vi "Check Overlay Settings.vi"(8 "error in (no error)":errorcluster, 9 "Mode":T2(ring), 10 "Overlay Settings":T3, 11 "Refnum in":T4) -> (0 "error out":errorcluster, 2 "Report Data":T1, 3 "Refnum out":T4)   [LabVIEW 2015]
uses:
  <vilib>/vision/Image Controls.llb/IMAQ Image.ctl
  Typedef/Last Mouse Position.ctl
  Typedef/Report Data.ctl
panel:
  out "accurate":dbl
  out "Dist.":dbl[][](array[numeric])
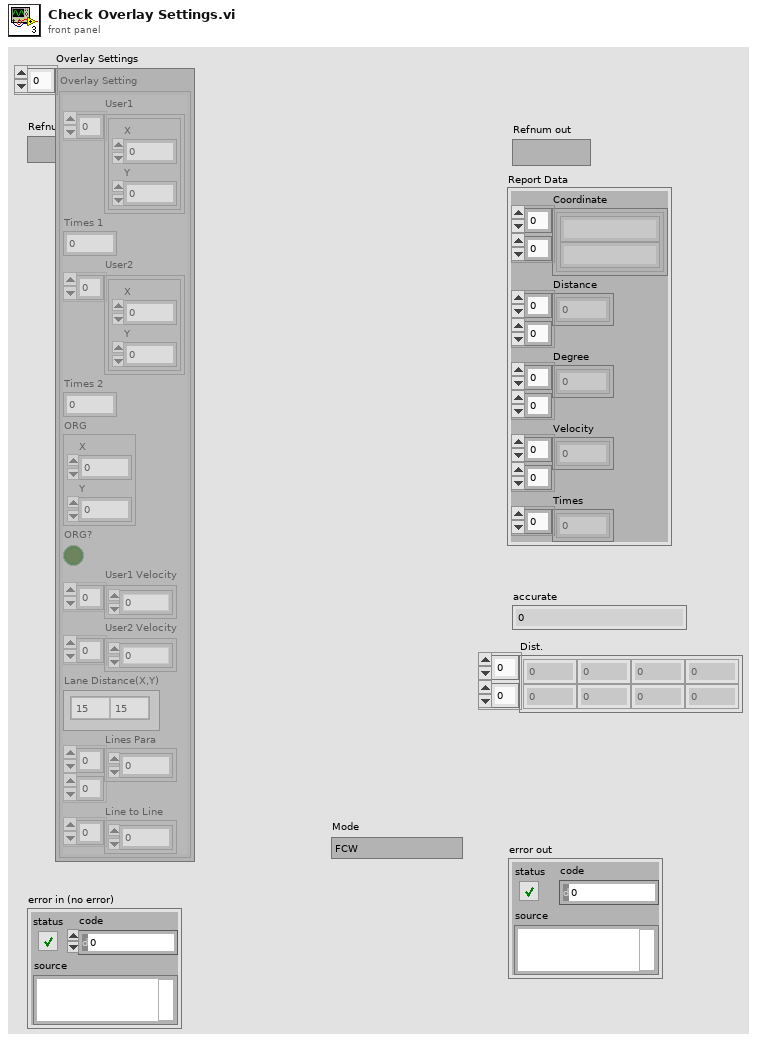
[diagram p1: front panel]
types:
  T1 = typedef "Report Data.ctl" = cluster{"Coordinate":cluster{string, string}[][], "Distance":dbl[][], "Degree":dbl[][], "Velocity":dbl[][], "Times":i32[]}
  T2 = enum16{"FCW", "BSD(Right)", "BSD(Left)", "RCTA(Right)", "RCTA(Left)", "DOW(Right)", "DOW(Left)"}
  T3 = typedef "Last Mouse Position.ctl" = cluster{"User1":cluster{"X":dbl, "Y":dbl}[], "Times 1":i32, "User2":cluster{"X":dbl, "Y":dbl}[], "Times 2":i32, "ORG":cluster{"X":dbl, "Y":dbl}, "ORG?":bool, "User1 Velocity":dbl[], "User2 Velocity":dbl[], "Lane Distance(X,Y)":cluster{"X":dbl, "Y":dbl}, "Lines Para":dbl[][], "Line to Line":dbl[]}[]
  T4 = typedef "IMAQ Image.ctl" = refnum<image>
  T5 = cluster{"User1":cluster{"X":dbl, "Y":dbl}[], "Times 1":i32, "User2":cluster{"X":dbl, "Y":dbl}[], "Times 2":i32, "ORG":cluster{"X":dbl, "Y":dbl}, "ORG?":bool, "User1 Velocity":dbl[], "User2 Velocity":dbl[], "Lane Distance(X,Y)":cluster{"X":dbl, "Y":dbl}, "Lines Para":dbl[][], "Line to Line":dbl[]}
  T6 = cluster{"Desired Font (Application)":enum16{"User-specified Font", "Application Font", "System Font", "Dialog Font"}, "[User-specified Font]":cluster{"Font Name":string, "Size":i16, "Strikeout?":bool, "Italic?":bool, "Underline?":bool, "Outline?":bool, "Shadow?":bool, "Bold?":bool, "Rotation Angle":dbl}, "Horizontal Alignment":i16, "Vertical Alignment":i16}
  T7 = cluster{cluster{string, string}[][], dbl[][], dbl[][], dbl[][], i32[]}
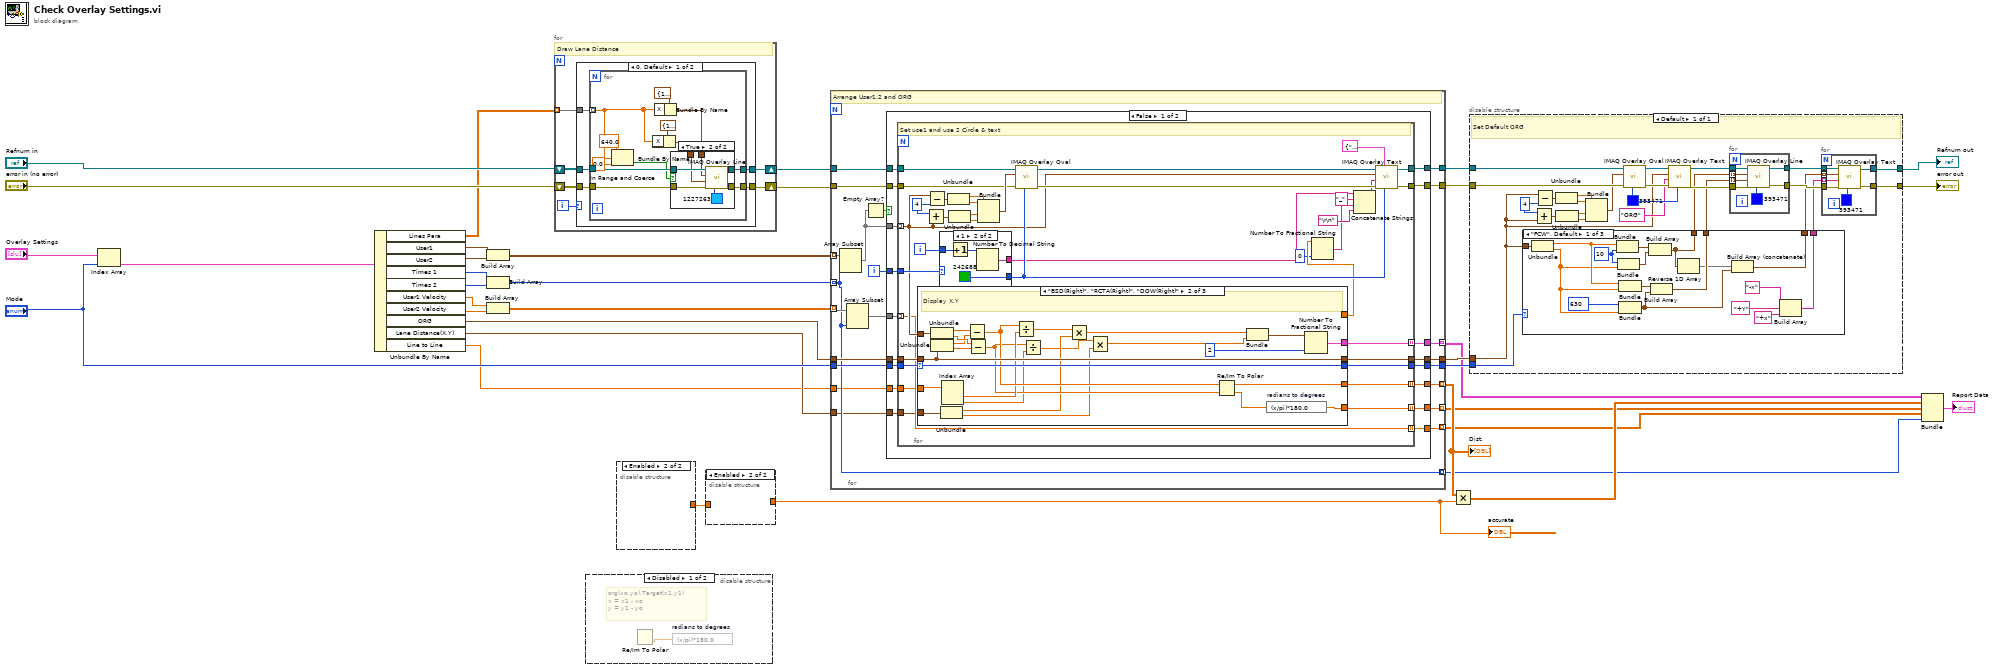
[diagram p0: block diagram]
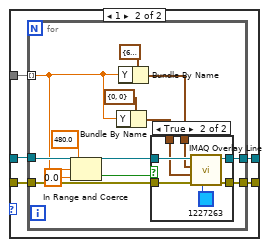
[diagram p3: hidden frame]
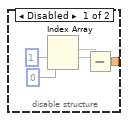
[diagram p5: hidden frame]
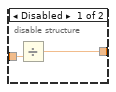
[diagram p6: hidden frame]
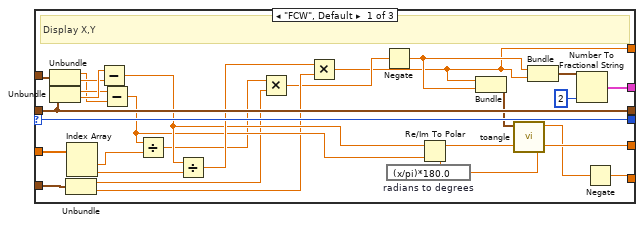
[diagram p8: hidden frame]
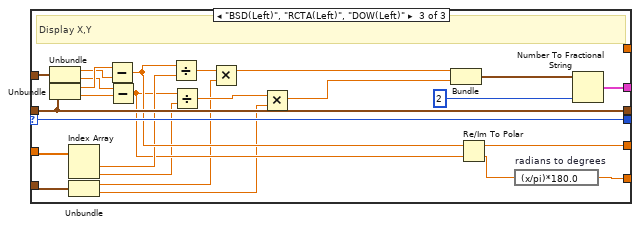
[diagram p9: hidden frame]
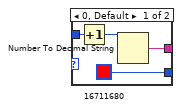
[diagram p10: hidden frame]
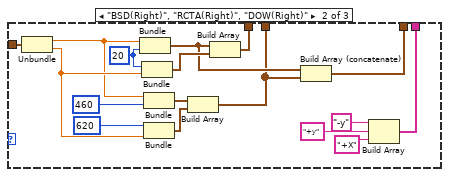
[diagram p12: hidden frame]
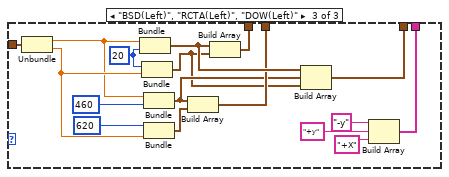
[diagram p13: hidden frame]
diagram:
  n1 = Index Array(array="Overlay Settings", index="Mode") -> (element=w18:T5)
  n2 = Unbundle By Name(w18) -> ("Lines Para"=w2:dbl[][], "User1"=w34:cluster{"X":dbl, "Y":dbl}[], "User2"=w35:cluster{"X":dbl, "Y":dbl}[], "Times 1"=w33:i32, "Times 2"=w31:i32, "User1 Velocity"=w12:dbl[], "User2 Velocity"=w13:dbl[], "ORG"=w11:cluster{"X":dbl, "Y":dbl}, "Lane Distance(X,Y)"=w7:cluster{"X":dbl, "Y":dbl}, "Line to Line"=w1:dbl[])
  n3 = Build Array(w34, w35) -> (w25:cluster{"X":dbl, "Y":dbl}[][])
  n4 = Build Array(w33, w31) -> (w32:i32[])
  n5 = Build Array(w12, w13) -> (w10:dbl[][])
  n6 = for {
    shift-right: [w40] -> w6
    shift-left: "Refnum in" -> [w41]
    shift-right: [w38] -> w5
    shift-left: "error in (no error)" -> [w39]
    tunnel: w2 -> [w36] mode=indexing
    i -> [w37]
    # "Draw Lane Distance"
    n7 = case shown="0, Default" w37 {
      tunnel: w41 -> [w46 w72]
      tunnel: [w45 w71] -> w40
      tunnel: w39 -> [w44 w70]
      tunnel: [w43 w69] -> w38
      tunnel: w36 -> [w42 w68]
      frame 0, Default {
        n8 = for {
          tunnel: w46 -> [w58]
          tunnel: [w57] -> w45
          tunnel: w44 -> [w56]
          tunnel: [w55] -> w43
          tunnel: w42 -> [w50] mode=indexing
          n9 = In Range and Coerce(upper limit=640.0, x=w50, lower limit=0.0) -> (In Range?=w49:bool)  [unwired: 1 out]
          n10 = Bundle By Name(cluster=cluster{"X":i32, "Y":i32} {"X"=113, "Y"=480} ("End Point"), "X"=w50) -> (w53:cluster{"X":i32, "Y":i32})
          n11 = Bundle By Name(cluster=cluster{"X":i32, "Y":i32} {"X"=113, "Y"=0} ("Start Point"), "X"=w50) -> (w54:cluster{"X":i32, "Y":i32})
          n12 = case shown="True" w49 {
            tunnel: w58 -> [w60 w66]
            tunnel: [w60 w65] -> w57
            tunnel: w56 -> [w59 w64]
            tunnel: [w59 w63] -> w55
            tunnel: w54 -> [_ w62]
            tunnel: w53 -> [_ w61]
            frame False {
            }
            frame True {
              n13 = call "IMAQ Overlay Line"("Color"=u32 1227263, "error in (no error)"=w64, "End Point"=w61, "Start Point"=w62, "Image"=w66) -> ("error out"=w63:errorcluster, "Image Out"=w65:T4)  [unwired: 5 in]
            }
          }
        }
      }
      frame 1 {
        n14 = for {
          tunnel: w72 -> [w84]
          tunnel: [w83] -> w71
          tunnel: w70 -> [w82]
          tunnel: [w81] -> w69
          tunnel: w68 -> [w76] mode=indexing
          n15 = In Range and Coerce(upper limit=480.0, x=w76, lower limit=0.0) -> (In Range?=w75:bool)  [unwired: 1 out]
          n16 = Bundle By Name(cluster=cluster{"X":i32, "Y":i32} {"X"=0, "Y"=0} ("End Point"), "Y"=w76) -> (w79:cluster{"X":i32, "Y":i32})
          n17 = Bundle By Name(cluster=cluster{"X":i32, "Y":i32} {"X"=640, "Y"=480} ("Start Point"), "Y"=w76) -> (w80:cluster{"X":i32, "Y":i32})
          n18 = case shown="True" w75 {
            tunnel: w84 -> [w86 w92]
            tunnel: [w86 w91] -> w83
            tunnel: w82 -> [w85 w90]
            tunnel: [w85 w89] -> w81
            tunnel: w80 -> [_ w88]
            tunnel: w79 -> [_ w87]
            frame False {
            }
            frame True {
              n19 = call "IMAQ Overlay Line"("Color"=u32 1227263, "error in (no error)"=w90, "End Point"=w87, "Start Point"=w88, "Image"=w92) -> ("error out"=w89:errorcluster, "Image Out"=w91:T4)  [unwired: 5 in]
            }
          }
        }
      }
    }
  }
  n20 = disable-structure shown="Disabled" {
    frame Disabled {
      # "org(xo,yo),Target(x1,y1)\nx = x1 - xo\ny = y1 - yo"
      n21 = Re/Im To Polar() -> (0:w94:dbl)  [unwired: 2 in, 1 out]
      n22 = expression code="(x/pi)*180.0" "radians to degrees"(w94) -> ()  [unwired: 1 out]
    }
    frame Enabled {
    }
  }
  n23 = disable-structure shown="Enabled" {
    disable-tunnel: [w95 _] -> w21
    frame Disabled {
      n24 = Index Array(index #1=1 ("index"), index #2=0 ("index")) -> (element #1=w97, element #2=w96)  [unwired: 1 in]
      n25 = Subtract(x=w97, y=w96) -> (x-y=w95:dbl)
    }
    frame Enabled {
    }
  }
  n26 = disable-structure shown="Enabled" {
    disable-tunnel: w21 -> [w101 _]
    disable-tunnel: [w100 _] -> w19
    frame Disabled {
      n27 = Divide(y=w101) -> (x/y=w100:dbl)  [unwired: 1 in]
    }
    frame Enabled {
    }
  }
  "accurate" <- w19
  n28 = for {
    tunnel: w6 -> [w122]
    tunnel: w32 -> [w106] mode=indexing
    tunnel: w25 -> [w117] mode=indexing
    tunnel: [w121] -> w29
    tunnel: w5 -> [w120]
    tunnel: [w119] -> w28
    tunnel: w11 -> [w114]
    tunnel: [w113] -> w24
    tunnel: "Mode" -> [w112]
    tunnel: [w111] -> w22
    tunnel: [w110] -> w17 mode=indexing
    tunnel: [w109] -> w14 mode=indexing
    tunnel: [w108] -> w20 mode=indexing
    tunnel: [w106] -> w8 mode=indexing
    tunnel: w10 -> [w107] mode=indexing
    tunnel: [w104] -> w9 mode=indexing
    tunnel: w1 -> [w103]
    tunnel: w7 -> [w102]
    i -> [w118]
    # "Arrange User1,2 and ORG"
    n29 = Array Subset(array=w117, length=w106) -> (w116:cluster{"X":dbl, "Y":dbl}[])  [unwired: 1 in]
    n30 = Array Subset(array=w107, length=w106) -> (w105:dbl[])  [unwired: 1 in]
    n31 = Empty Array?(array=w116) -> (empty?=w115:bool)
    n32 = case shown="False" w115 {
      tunnel: w122 -> [w139 w266]
      tunnel: [w138 w266] -> w121
      tunnel: w120 -> [w137 w265]
      tunnel: [w136 w265] -> w119
      tunnel: w118 -> [w135 _]
      tunnel: w116 -> [w134 _]
      tunnel: w114 -> [w133 w264]
      tunnel: [w132 w264] -> w113
      tunnel: w112 -> [w131 w263]
      tunnel: [w130 w263] -> w111
      tunnel: [w129 _] -> w110
      tunnel: [w128 _] -> w109
      tunnel: [w127 _] -> w108
      tunnel: w105 -> [w126 _]
      tunnel: [w125 _] -> w104
      tunnel: w103 -> [w124 _]
      tunnel: w102 -> [w123 _]
      frame False {
        n33 = for {
          tunnel: w139 -> [w175]
          tunnel: w134 -> [w155] mode=indexing
          tunnel: w135 -> [w165]
          tunnel: [w163] -> w138
          tunnel: w137 -> [w162]
          tunnel: [w160] -> w136
          tunnel: w133 -> [w157]
          tunnel: [w154] -> w132
          tunnel: w131 -> [w158]
          tunnel: [w156] -> w130
          tunnel: [w153] -> w129 mode=indexing
          tunnel: [w151] -> w128 mode=indexing
          tunnel: [w152] -> w127 mode=indexing
          tunnel: w126 -> [w149] mode=indexing
          tunnel: [w149] -> w125 mode=indexing
          tunnel: w124 -> [w148]
          tunnel: w123 -> [w147]
          i -> [w159]
          w167 = 4
          # "Set use1 and use 2 Circle & text"
          n34 = case shown="\"BSD(Right)\", \"RCTA(Right)\", \"DOW(Right)\"" w158 {
            selector: w158 -> [w204 w229 w254]
            tunnel: w157 -> [w203 w227 w252]
            tunnel: [w204 w229 w254] -> w156
            tunnel: w155 -> [w183 w228 w253]
            tunnel: [w203 w227 w252] -> w154
            tunnel: [w202 w225 w250] -> w153
            tunnel: [w179 w219 w244] -> w151
            tunnel: [w196 w218 w243] -> w152
            tunnel: w148 -> [w195 w217 w240]
            tunnel: w147 -> [w187 w210 w234]
            tunnel: [w176 _ _] -> w144
            frame "FCW", Default {
              # "Display X,Y"
              n35 = Unbundle(w183) -> ("X"=w198:dbl, "Y"=w200:dbl)
              n36 = Unbundle(w203) -> ("X"=w199:dbl, "Y"=w201:dbl)
              n37 = Unbundle(w187) -> ("X"=w186:dbl, "Y"=w185:dbl)
              n38 = Index Array(array=w195) -> (element #1=w188:dbl, element #2=w189:dbl)  [unwired: 2 in]
              n39 = Subtract(x=w201, y=w200) -> (x-y=w193:dbl)
              n40 = Subtract(x=w199, y=w198) -> (x-y=w192:dbl)
              n41 = Divide(x=w192, y=w188) -> (x/y=w191:dbl)
              n42 = Divide(x=w193, y=w189) -> (x/y=w194:dbl)
              n43 = Multiply(x=w191, y=w186) -> (x*y=w180:dbl)
              n44 = Multiply(x=w194, y=w185) -> (x*y=w176:dbl)
              n45 = Negate(x=w180) -> (-x=w177:dbl)
              n46 = Re/Im To Polar(2:w192, 3:w193) -> (0:w197:dbl, 1:w196:dbl)
              n47 = expression code="(x/pi)*180.0" "radians to degrees"(w197) -> (w182:dbl)
              n48 = Bundle(w176, w177) -> (w184:cluster{dbl, dbl})  [unwired: 1 in]
              n49 = call "toangle.vi"("Numeric"=w182, "number"=w184) -> ("atan2(y,x)"=w178:dbl)  [unwired: 9 in]
              n50 = Bundle(w177, w176) -> (w181:cluster{dbl, dbl})  [unwired: 1 in]
              n51 = Number To Fractional String(number=w181, precision (6)=i16 2) -> (F-format string=w202:cluster{string, string})  [unwired: 2 in]
              n52 = Negate(x=w178) -> (-x=w179:dbl)
            }
            frame "BSD(Right)", "RCTA(Right)", "DOW(Right)" {
              # "Display X,Y"
              n53 = Unbundle(w228) -> ("X"=w224:dbl, "Y"=w222:dbl)
              n54 = Unbundle(w227) -> ("X"=w221:dbl, "Y"=w223:dbl)
              n55 = Unbundle(w210) -> ("X"=w208:dbl, "Y"=w205:dbl)
              n56 = Index Array(array=w217) -> (element #1=w214:dbl, element #2=w212:dbl)  [unwired: 2 in]
              n57 = Subtract(x=w224, y=w221) -> (x-y=w215:dbl)
              n58 = Subtract(x=w222, y=w223) -> (x-y=w213:dbl)
              n59 = Divide(x=w215, y=w214) -> (x/y=w216:dbl)
              n60 = Divide(x=w213, y=w212) -> (x/y=w206:dbl)
              n61 = Multiply(x=w216, y=w208) -> (x*y=w209:dbl)
              n62 = Multiply(x=w206, y=w205) -> (x*y=w207:dbl)
              n63 = Re/Im To Polar(2:w213, 3:w215) -> (0:w220:dbl, 1:w218:dbl)
              n64 = Bundle(w209, w207) -> (w226:cluster{dbl, dbl})  [unwired: 1 in]
              n65 = expression code="(x/pi)*180.0" "radians to degrees"(w220) -> (w219:dbl)
              n66 = Number To Fractional String(number=w226, precision (6)=i16 2) -> (F-format string=w225:cluster{string, string})  [unwired: 2 in]
            }
            frame "BSD(Left)", "RCTA(Left)", "DOW(Left)" {
              # "Display X,Y"
              n67 = Unbundle(w253) -> ("X"=w248:dbl, "Y"=w247:dbl)
              n68 = Unbundle(w252) -> ("X"=w249:dbl, "Y"=w246:dbl)
              n69 = Index Array(array=w240) -> (element #1=w239:dbl, element #2=w237:dbl)  [unwired: 2 in]
              n70 = Unbundle(w234) -> ("X"=w232:dbl, "Y"=w230:dbl)
              n71 = Subtract(x=w249, y=w248) -> (x-y=w241:dbl)
              n72 = Subtract(x=w247, y=w246) -> (x-y=w238:dbl)
              n73 = Divide(x=w241, y=w239) -> (x/y=w242:dbl)
              n74 = Divide(x=w238, y=w237) -> (x/y=w236:dbl)
              n75 = Multiply(x=w242, y=w232) -> (x*y=w233:dbl)
              n76 = Multiply(x=w236, y=w230) -> (x*y=w231:dbl)
              n77 = Bundle(w233, w231) -> (w251:cluster{dbl, dbl})  [unwired: 1 in]
              n78 = Re/Im To Polar(2:w238, 3:w241) -> (0:w245:dbl, 1:w243:dbl)
              n79 = expression code="(x/pi)*180.0" "radians to degrees"(w245) -> (w244:dbl)
              n80 = Number To Fractional String(number=w251, precision (6)=i16 2) -> (F-format string=w250:cluster{string, string})  [unwired: 2 in]
            }
          }
          n81 = Add(x=w167, y=w155) -> (x+y=w171:cluster{"X":dbl, "Y":dbl})
          n82 = Subtract(x=w155, y=w167) -> (x-y=w169:cluster{"X":dbl, "Y":dbl})
          n83 = case shown="1" w165 {
            tunnel: [u32 16711680 ("Color") u32 242688 ("Color")] -> w164
            tunnel: w159 -> [w256 w260]
            tunnel: [w255 w259] -> w141
            frame 0, Default {
              n84 = Increment(x=w256) -> (x+1=w257:i32)
              n85 = Number To Decimal String(number=w257) -> (decimal integer string=w255:string)  [unwired: 1 in]
            }
            frame 1 {
              n86 = Increment(x=w260) -> (x+1=w261:i32)
              n87 = Number To Decimal String(number=w261) -> (decimal integer string=w259:string)  [unwired: 1 in]
            }
          }
          n88 = Unbundle(w169) -> ("X"=w168:dbl, "Y"=w170:dbl)
          n89 = Unbundle(w171) -> ("X"=w172:dbl, "Y"=w173:dbl)
          n90 = Bundle("X"=w168, "Y"=w170, "X"=w172, "Y"=w173) -> (w166:cluster{"X":dbl, "Y":dbl, "X":dbl, "Y":dbl})  [unwired: 1 in]
          n91 = call "IMAQ Overlay Oval"("Color"=w164, "error in (no error)"=w162, "Bounding Rectangle"=w166, "Image"=w175) -> ("error out"=w161:errorcluster, "Image Out"=w174:T4)  [unwired: 6 in]
          n92 = Number To Fractional String(number=w144, precision (6)=i16 0) -> (F-format string=w143:string)  [unwired: 2 in]
          n93 = Concatenate Strings(w141, "_" ("string"), w143, "\r\n") -> (w150:string)
          n94 = call "IMAQ Overlay Text"("Text Color (black)"=w164, "Font, Size & Style"=T6 {"Desired Font (Application)"=enum."Application Font", "[User-specified Font]"={"Font Name"="", "Size"=12, "Strikeout?"=FALSE, "Italic?"=FALSE, "Underline?"=FALSE, "Outline?"=FALSE, "Shadow?"=FALSE, "Bold?"=FALSE, "Rotation Angle"=0.0}, "Horizontal Alignment"=0, "Vertical Alignment"=0}, "error in (no error)"=w161, "String"=w150, "Origin"=w155, "Image"=w174) -> ("error out"=w160:errorcluster, "Image Out"=w163:T4)  [unwired: 4 in]
        }
      }
      frame True {
      }
    }
  }
  "Dist." <- w20
  n95 = Multiply(x=w20, y=w19) -> (x*y=w16:dbl[][])
  n96 = disable-structure shown="Default" {
    disable-tunnel: w29 -> [w292]
    disable-tunnel: w28 -> [w291]
    disable-tunnel: [w290] -> w27
    disable-tunnel: [w289] -> w26
    disable-tunnel: w24 -> [w267]
    disable-tunnel: w22 -> [w288]
    frame Enabled {
      w278 = u32 393471 ("Color")
      w280 = 4
      # "Set Default ORG"
      n97 = case shown="\"FCW\", Default" w288 {
        tunnel: w267 -> [w300 w333 w350]
        tunnel: [w303 w320 w338] -> w273
        tunnel: [w311 w317 w336] -> w272
        tunnel: [w307 w323 w341] -> w269
        tunnel: [w306 w322 w340] -> w268
        frame "FCW", Default {
          w314 = 10
          n98 = Unbundle(w300) -> ("X"=w315:dbl, "Y"=w301:dbl)
          n99 = Bundle("X"=w315, w314) -> (w304:cluster{"X":dbl, i32})  [unwired: 1 in]
          n100 = Bundle(w314, "Y"=w301) -> (w312:cluster{i32, "Y":dbl})  [unwired: 1 in]
          n101 = Bundle("X"=w315, "Y"=w301) -> (w313:cluster{"X":dbl, "Y":dbl})  [unwired: 1 in]
          n102 = Bundle(630, "Y"=w301) -> (w305:cluster{i32, "Y":dbl})  [unwired: 1 in]
          n103 = Build Array(w304, w312) -> (w303:cluster{"X":dbl, "Y":dbl}[])
          n104 = Build Array(w313, w305) -> (w311:cluster{"X":dbl, "Y":dbl}[])
          n105 = Reverse 1D Array(array=w303) -> (reversed array=w302:cluster{"X":dbl, "Y":dbl}[])
          n106 = Build Array (concatenate)(w302, w305) -> (w306:cluster{"X":dbl, "Y":dbl}[])
          n107 = Build Array("-x", "+Y", "+x") -> (w307:string[])
        }
        frame "BSD(Right)", "RCTA(Right)", "DOW(Right)" {
          w328 = 20
          n108 = Unbundle(w333) -> ("X"=w330:dbl, "Y"=w332:dbl)
          n109 = Bundle("X"=w330, w328) -> (w318:cluster{"X":dbl, i32})  [unwired: 1 in]
          n110 = Bundle(w328, "Y"=w332) -> (w319:cluster{i32, "Y":dbl})  [unwired: 1 in]
          n111 = Bundle("X"=w330, 460) -> (w327:cluster{"X":dbl, i32})  [unwired: 1 in]
          n112 = Bundle(620, "Y"=w332) -> (w321:cluster{i32, "Y":dbl})  [unwired: 1 in]
          n113 = Build Array(w327, w321) -> (w317:cluster{"X":dbl, "Y":dbl}[])
          n114 = Build Array(w318, w319) -> (w320:cluster{"X":dbl, "Y":dbl}[])
          n115 = Build Array (concatenate)(w318, w317) -> (w322:cluster{"X":dbl, "Y":dbl}[])
          n116 = Build Array("-y", "+y", "+X") -> (w323:string[])
        }
        frame "BSD(Left)", "RCTA(Left)", "DOW(Left)" {
          w345 = 20
          n117 = Unbundle(w350) -> ("X"=w347:dbl, "Y"=w349:dbl)
          n118 = Bundle("X"=w347, w345) -> (w337:cluster{"X":dbl, i32})  [unwired: 1 in]
          n119 = Bundle(w345, "Y"=w349) -> (w334:cluster{i32, "Y":dbl})  [unwired: 1 in]
          n120 = Bundle("X"=w347, 460) -> (w335:cluster{"X":dbl, i32})  [unwired: 1 in]
          n121 = Bundle(620, "Y"=w349) -> (w339:cluster{i32, "Y":dbl})  [unwired: 1 in]
          n122 = Build Array(w335, w339) -> (w336:cluster{"X":dbl, "Y":dbl}[])
          n123 = Build Array(w337, w334) -> (w338:cluster{"X":dbl, "Y":dbl}[])
          n124 = Build Array(w337, w335, w334) -> (w340:cluster{"X":dbl, "Y":dbl}[])
          n125 = Build Array("-y", "+y", "+X") -> (w341:string[])
        }
      }
      n126 = Add(x=w280, y=w267) -> (x+y=w284:cluster{"X":dbl, "Y":dbl})
      n127 = Subtract(x=w267, y=w280) -> (x-y=w282:cluster{"X":dbl, "Y":dbl})
      n128 = Unbundle(w282) -> ("X"=w281:dbl, "Y"=w283:dbl)
      n129 = Unbundle(w284) -> ("X"=w285:dbl, "Y"=w286:dbl)
      n130 = Bundle("X"=w281, "Y"=w283, "X"=w285, "Y"=w286) -> (w279:cluster{"X":dbl, "Y":dbl, "X":dbl, "Y":dbl})  [unwired: 1 in]
      n131 = call "IMAQ Overlay Oval"("Color"=w278, "error in (no error)"=w291, "Bounding Rectangle"=w279, "Image"=w292) -> ("error out"=w277:errorcluster, "Image Out"=w287:T4)  [unwired: 6 in]
      n132 = call "IMAQ Overlay Text"("Text Color (black)"=w278, "error in (no error)"=w277, "String"="ORG", "Origin"=w267, "Image"=w287) -> ("error out"=w274:errorcluster, "Image Out"=w275:T4)  [unwired: 5 in]
      n133 = for {
        tunnel: w275 -> [w357]
        tunnel: [w356] -> w271
        tunnel: w274 -> [w355]
        tunnel: [w354] -> w270
        tunnel: w273 -> [w353] mode=indexing
        tunnel: w272 -> [w352] mode=indexing
        n134 = call "IMAQ Overlay Line"("Color"=u32 393471, "error in (no error)"=w355, "End Point"=w352, "Start Point"=w353, "Image"=w357) -> ("error out"=w354:errorcluster, "Image Out"=w356:T4)  [unwired: 5 in]
      }
      n135 = for {
        tunnel: w271 -> [w299]
        tunnel: w270 -> [w298]
        tunnel: [w297] -> w290
        tunnel: [w296] -> w289
        tunnel: w269 -> [w295] mode=indexing
        tunnel: w268 -> [w294] mode=indexing
        n136 = call "IMAQ Overlay Text"("Text Color (black)"=u32 393471 ("Color"), "error in (no error)"=w298, "String"=w295, "Origin"=w294, "Image"=w299) -> ("error out"=w297:errorcluster, "Image Out"=w296:T4)  [unwired: 5 in]
      }
    }
  }
  "error out" <- w27
  "Refnum out" <- w26
  n137 = Bundle(w17, w16, w14, w9, w8) -> (→"Report Data":T7)  [unwired: 1 in]
